vi "FTW-ScheduledJobset-AddOrReplace.vi"(0 "FTW Scheduled Jobset":refnum<class "FTW-ScheduledJob.lvclass">[](array[class]), 5 "FTW Scheduled Job":refnum<class "FTW-ScheduledJob.lvclass">, 7 "Replace if already exists":bool=TRUE, 11 "error in":errorcluster) -> (4 "FTW Scheduled Jobset out":refnum<class "FTW-ScheduledJob.lvclass">[](array[class]), 15 "error out":errorcluster)   [LabVIEW 2015, in "FTW-ScheduledJob.lvclass"]
uses:
  FTW-ScheduledJob.lvclass
  FTW-ScheduledJob.lvclass/FTW-ScheduledJob.ctl
panel:
  # "Inputs"
  # "Outputs"
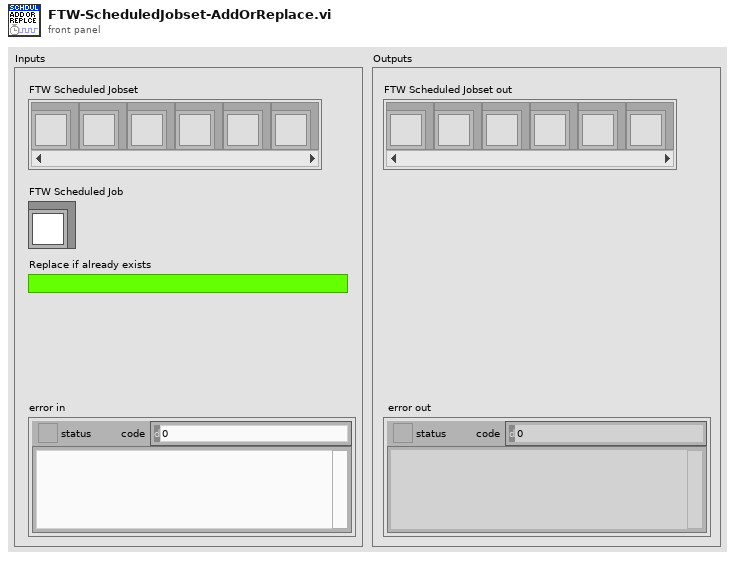
[diagram p1: front panel]
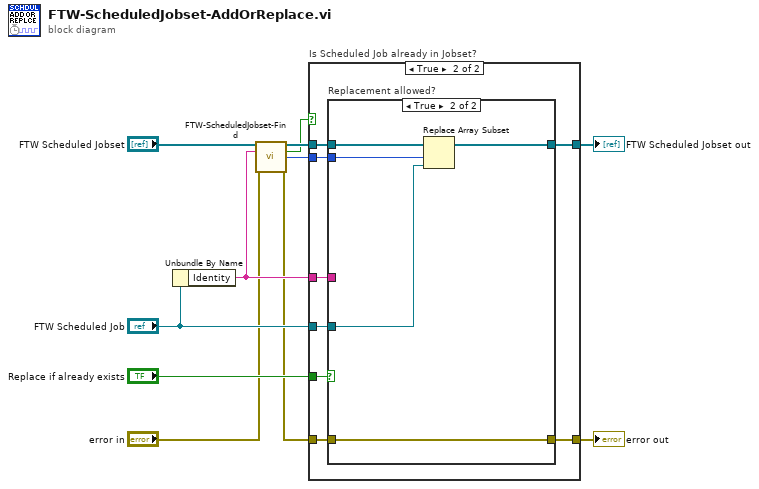
[diagram p0: block diagram]
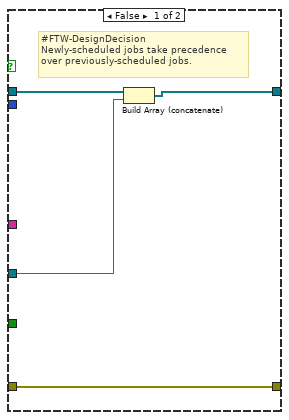
[diagram p2: hidden frame]
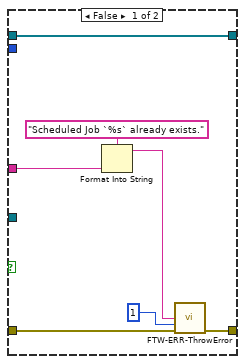
[diagram p3: hidden frame]
diagram:
  n1 = Unbundle By Name("FTW Scheduled Job") -> ("Identity"=w5:string)
  n2 = call "FTW-ScheduledJobset-Find.vi"("FTW Scheduled Jobset"="FTW Scheduled Jobset", "Identity"=w5, "error in"="error in") -> ("FTW Scheduled Jobset out"=w6:refnum<class "FTW-ScheduledJob.lvclass">[], "Found?"=w2:bool, "Index"=w1:i32, "error out"=w3:errorcluster)  [unwired: 9 in]
  n3 = case "Is Scheduled Job already in Jobset?" shown="True" w2 {
    tunnel: [w14 w19] -> w11
    tunnel: w6 -> [w15 w18]
    tunnel: [w12 w20] -> w10
    tunnel: w3 -> [w12 w21]
    tunnel: "FTW Scheduled Job" -> [w13 w16]
    tunnel: w5 -> [_ w23]
    tunnel: w1 -> [_ w17]
    tunnel: "Replace if already exists" -> [_ w22]
    frame False {
      # "#FTW-DesignDecision\nNewly-scheduled jobs take precedence\nover previously-scheduled jobs."
      n4 = Build Array (concatenate)(w15, w13) -> (w14:refnum<class "FTW-ScheduledJob.lvclass">[])
    }
    frame True {
      n5 = case "Replacement allowed?" shown="True" w22 {
        tunnel: w23 -> [w30 _]
        tunnel: w21 -> [w28 w35]
        tunnel: [w27 w35] -> w20
        tunnel: [w25 w33] -> w19
        tunnel: w18 -> [w25 w34]
        tunnel: w17 -> [_ w32]
        tunnel: w16 -> [_ w31]
        frame False {
          n6 = Format Into String(format string="Scheduled Job `%s` already exists.", w30) -> (resulting string=w26:string)  [unwired: 2 in, 1 out]
          n7 = call "FTW-ERR-ThrowError.vi"("Error Message"=w26, "Error Code"=1, "error in"=w28) -> ("error out"=w27:errorcluster)  [unwired: 12 in]
        }
        frame True {
          n8 = Replace Array Subset(array=w34, new element=w31, index=w32) -> (w33:refnum<class "FTW-ScheduledJob.lvclass">[])
        }
      }
    }
  }
  "FTW Scheduled Jobset out" <- w11
  "error out" <- w10
